vi "IndexingTypes.vi"() -> ()   [LabVIEW 2014]
panel:
  out "Concatenating":sgl[](array[numeric])
  out "Indexing array out":sgl[][](array[numeric])
  out "Last Value":sgl
  in  "Loop Iterations":i32=5
  in  "Non-indexing Array":sgl[](array[numeric])
  out "Last Value Array out":sgl[](array[numeric])
  out "Indexing array out":sgl[](array[numeric])
  in  "Indexing Array":sgl[](array[numeric])
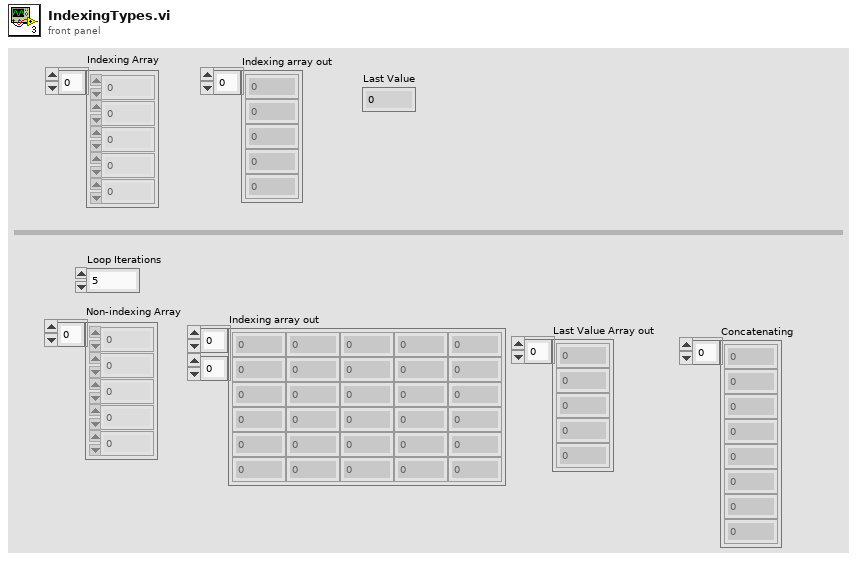
[diagram p1: front panel]
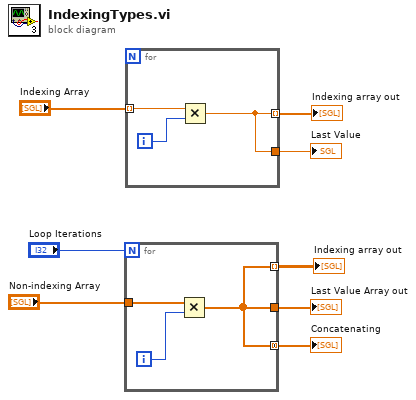
[diagram p0: block diagram]
diagram:
  n1 = for {
    N: "Loop Iterations" -> [_]
    tunnel: "Non-indexing Array" -> [w11]
    tunnel: [w9] -> w7
    tunnel: [w9] -> w2 mode=indexing
    tunnel: [w9] -> w1 mode=concatenating
    i -> [w10]
    n2 = Multiply(x=w11, y=w10) -> (x*y=w9:sgl[])
  }
  "Last Value Array out" <- w7
  "Indexing array out" <- w2
  "Concatenating" <- w1
  n3 = for {
    tunnel: "Indexing Array" -> [w14] mode=indexing
    tunnel: [w12] -> w8 mode=indexing
    tunnel: [w12] -> w3
    i -> [w13]
    n4 = Multiply(x=w14, y=w13) -> (x*y=w12:sgl)
  }
  "Indexing array out" <- w8
  "Last Value" <- w3
